vi "PDCGetPictureData.vi"(5 "Resolution":cluster{"Width":u32, "Height":u32}, 6 "Data(8Bit)":u8[](array[numeric]), 7 "ColorType":enum16{"MONO", "COLOR"}(ring)) -> (3 "ImageData":T1)   [LabVIEW 2015]
uses:
  <vilib>/picture/picture.llb/imagedata.ctl
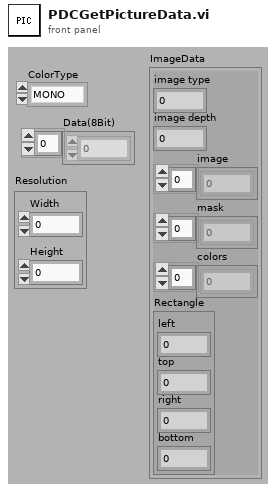
[diagram p1: front panel]
types:
  T1 = typedef "imagedata.ctl" = cluster{"image type":i32, "image depth":i32, "image":u8[], "mask":u8[], "colors":u32[], "Rectangle":cluster{"left":i16, "top":i16, "right":i16, "bottom":i16}}
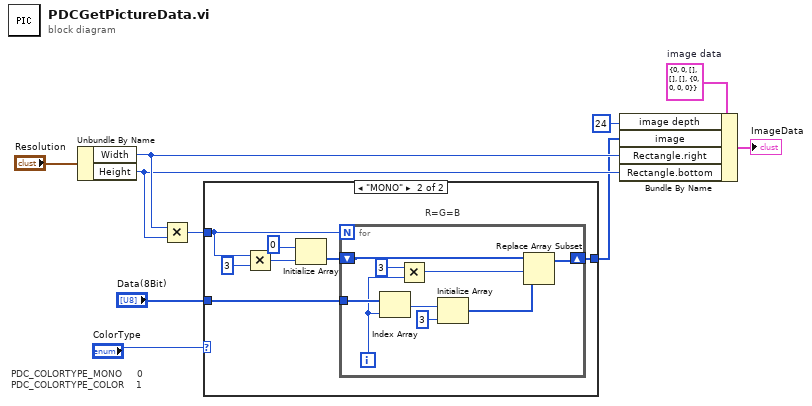
[diagram p0: block diagram]
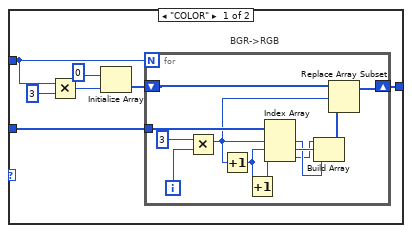
[diagram p2: hidden frame]
diagram:
  w2 = T1 {"image type"=0, "image depth"=0, "image"=[], "mask"=[], "colors"=[], "Rectangle"={"left"=0, "top"=0, "right"=0, "bottom"=0}}  # image data
  # "PDC_COLORTYPE_MONO\t\t\t\t\t0\nPDC_COLORTYPE_COLOR\t\t\t\t1"
  n1 = Unbundle By Name("Resolution") -> ("Width"=w6:u32, "Height"=w5:u32)
  n2 = Multiply(x=w6, y=w5) -> (x*y=w7:u32)
  n3 = case shown="\"MONO\"" "ColorType" {
    tunnel: w7 -> [w16 w35]
    tunnel: [w12 w31] -> w4
    tunnel: "Data(8Bit)" -> [w11 w30]
    frame "COLOR" {
      # "BGR->RGB"
      n4 = Multiply(x=w16, y=3) -> (x*y=w14:u32)
      n5 = Initialize Array(u8 0, w14) -> (w13:u8[])
      n6 = for {
        N: w16 -> [_]
        shift-right: [w20] -> w12
        shift-left: w13 -> [w21]
        tunnel: w11 -> [w29]
        i -> [w24]
        n7 = Multiply(x=3, y=w24) -> (x*y=w18:i32)
        n8 = Increment(x=w18) -> (x+1=w23:i32)
        n9 = Increment(x=w23) -> (x+1=w22:i32)
        n10 = Index Array(array=w29, index #1=w18, index #2=w23, index #3=w22) -> (element #1=w27:u8, element #2=w28:u8, element #3=w26:u8)
        n11 = Build Array(w26, w28, w27) -> (w19:u8[])
        n12 = Replace Array Subset(array=w21, new element=w19, index=w18) -> (w20:u8[])
      }
    }
    frame "MONO" {
      # "R=G=B"
      n13 = Multiply(x=w35, y=3) -> (x*y=w33:u32)
      n14 = Initialize Array(u8 0, w33) -> (w32:u8[])
      n15 = for {
        N: w35 -> [_]
        shift-right: [w42] -> w31
        shift-left: w32 -> [w43]
        tunnel: w30 -> [w45]
        i -> [w40]
        n16 = Index Array(array=w45, index=w40) -> (element=w39:u8)
        n17 = Multiply(x=3, y=w40) -> (x*y=w41:i32)
        n18 = Initialize Array(w39, 3 ("次元サイズ")) -> (w37:u8[])
        n19 = Replace Array Subset(array=w43, new element=w37, index=w41) -> (w42:u8[])
      }
    }
  }
  n20 = Bundle By Name(cluster=w2, "image depth"=24, "image"=w4, "Rectangle.right"=w6, "Rectangle.bottom"=w5) -> (→"ImageData":T1)
